vi "Insert Start Message.vi"(8 "error in (no error)":errorcluster, 10 "Start Time":timestamp, 11 "TimeStamper in":refnum<class "TimeStamper.lvclass">) -> (0 "error out":errorcluster, 3 "TimeStamper out":refnum<class "TimeStamper.lvclass">)   [LabVIEW 2010, in "TimeStamper.lvclass"]
uses:
  TimeStamper.lvclass
  Database/SessionPrimary.ctl
  AcquistionObject/AcquistionObject.lvclass
  TimeStamper.lvclass/TimeStamper.ctl
  <vilib>/addons/database/NI_Database_API.lvlib
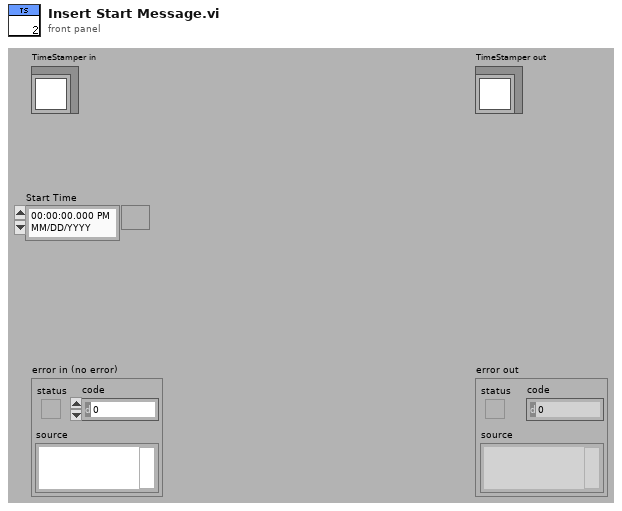
[diagram p1: front panel]
types:
  T1 = typedef "SessionPrimary.ctl" = cluster{"setup":u8, "session_start_time":dbl}
  T2 = cluster{"setup":u8, "subject":string, "experimenter":string, "session_start_time":dbl, "session_path":path}
  T3 = typedef "NI_Database_API.lvlib/Conn ObjectReference.ctl" = refnum<k1>
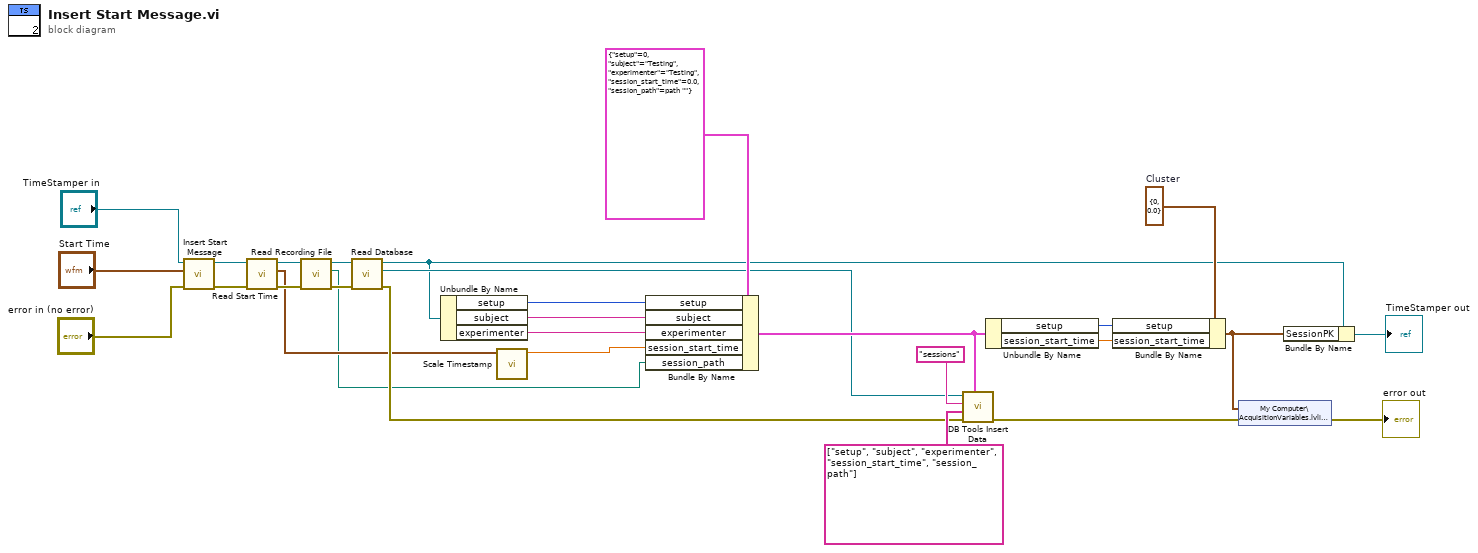
[diagram p0: block diagram]
diagram:
  w23 = T1 {"setup"=0, "session_start_time"=0.0}  # Cluster
  n1 = call-parent "Insert Start Message.vi"("error in (no error)"="error in (no error)", "Start Time"="Start Time", "AcquistionObject in"="TimeStamper in") -> ("error out"=w14:errorcluster, "AcquistionObject out"=w5:refnum<class "TimeStamper.lvclass">)  [unwired: 7 in]
  n2 = call-dynamic "Read Start Time.vi"("error in (no error)"=w14, "AcquistionObject in"=w5) -> ("error out"=w13:errorcluster, "Start Time"=w3:timestamp, "AcquistionObject out"=w7:refnum<class "TimeStamper.lvclass">)  [unwired: 7 in]
  n3 = call-dynamic "Read Recording File.vi"("error in (no error)"=w13, "AcquistionObject in"=w7) -> ("error out"=w12:errorcluster, "Recording File"=w1:path, "AcquistionObject out"=w6:refnum<class "TimeStamper.lvclass">)  [unwired: 7 in]
  n4 = call-dynamic "Read Database.vi"("error in (no error)"=w12, "AcquistionObject in"=w6) -> ("error out"=w11:errorcluster, "reference"=w15:T3)  [unwired: 7 in, 1 out]
  n5 = Unbundle By Name(w5) -> ("setup"=w18:u8, "subject"=w17:string, "experimenter"=w16:string)
  n6 = call "Scale Timestamp.vi"("Time Stamp"=w3) -> ("Scaled timestamp"=w2:dbl)  [unwired: 10 in]
  n7 = Bundle By Name(cluster=T2 {"setup"=0, "subject"="Testing", "experimenter"="Testing", "session_start_time"=0.0, "session_path"=path ""} ("Cluster"), "setup"=w18, "subject"=w17, "experimenter"=w16, "session_start_time"=w2, "session_path"=w1) -> (w22:T2)
  n8 = call <vilib>:"DB Tools Insert Data.vi"("data"=w22, "error in (no error)"=w11, "columns"=string[] ["setup", "subject", "experimenter", "session_start_time", "session_path"], "table"="sessions", "connection reference"=w15) -> ("error out"=w19:errorcluster)  [unwired: 5 in, 1 out]
  n9 = Unbundle By Name(w22) -> ("setup"=w21:u8, "session_start_time"=w20:dbl)
  n10 = Bundle By Name(cluster=w23, "setup"=w21, "session_start_time"=w20) -> (w10:T1)
  n11 = shared-variable "My Computer\\AcquisitionVariables.lvlib\\SessionPK"(w10, error in=w19) -> (error out=→"error out":errorcluster)
  n12 = Bundle By Name(cluster=w5, "SessionPK"=w10) -> (→"TimeStamper out":refnum<class "TimeStamper.lvclass">)
